vi "Maj.vi"(9 "z":u64, 10 "y":u64, 11 "x":u64) -> (3 "Maj":u64)   [LabVIEW 2020, in "NI_SHA-512.lvclass"]
doc: "Computes the function Maj(x, y, z) as defined in the SHA-2 specification."
uses:
  <vilib>/security/Message Digest/SHA-2/SHA-512/NI_SHA-512.lvclass
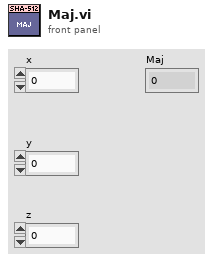
[diagram p1: front panel]
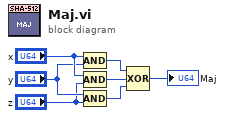
[diagram p0: block diagram]
diagram:
  n1 = Compound Arithmetic op=AND("x", "y") -> (w7:u64)
  n2 = Compound Arithmetic op=AND("x", "z") -> (w6:u64)
  n3 = Compound Arithmetic op=AND("y", "z") -> (w5:u64)
  n4 = Compound Arithmetic op=XOR(w7, w6, w5) -> (→"Maj":u64)
